vi "Lab3_6Var.vi"() -> ()   [LabVIEW 2022 SP3]
uses:
  f8ae16d3-e3a0-4295-90ca-0268b21e4943.vi
  <vilib>/Comparison/Less/Less Functor/Less Functor.lvclass
panel:
  in  "String":string
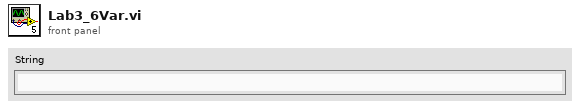
[diagram p1: front panel]
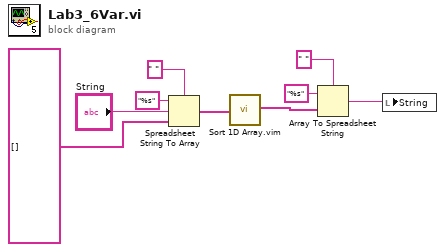
[diagram p0: block diagram]
diagram:
  n1 = Spreadsheet String To Array(delimiter (Tab)=" ", format string="%s", spreadsheet string="String", array type (2D Dbl)=string[] []) -> (array=w5:string[])
  n2 = call "Sort 1D Array.vim"("unsorted array"=w5) -> ("sorted array"=w4:string[])  [unwired: 10 in]
  n3 = Array To Spreadsheet String(delimiter (Tab)=" ", array=w4, 3:"%s" ("format string")) -> (spreadsheet string=w1:string)
  n4 = local write "String"(w1) -> ()
